vi "RSZVB Set Generator Step Attenuators.vi"(7 "Attenuation Factor (0.0)":dbl format="%^.3e", 8 "error in (no error)":errorcluster {"code" format="%.0x"}, 9 "Port (1)":i32=1, 10 "Channel (1)":i32=1, 11 "VISA session":refnum<visa-resource-name>) -> (0 "error out":errorcluster {"code" format="%.0x"}, 3 "dup VISA session":refnum<visa-resource-name>)   [LabVIEW 2011]
doc: "This VI sets a fixed attenuation factor for the generated wave at test port no. <Pt>. \n\nNote(s):\n\n(1) This VI can be used only with R&S ZVA and ZVB instruments.\n\nRemote-control command(s):\nSOURce<Ch>:POWer<Pt>:ATTenuation <numeric_value>"
uses:
  _utility/RSZVB Global Data.vi
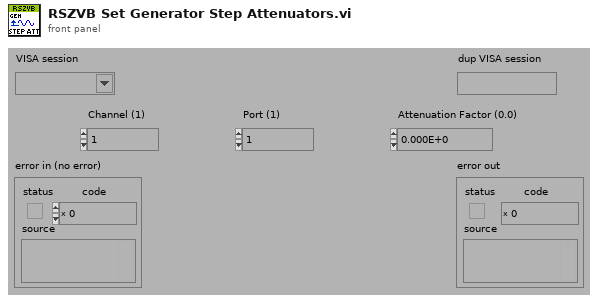
[diagram p1: front panel]
types:
  T1 = cluster{"Error Checking (T: On)":bool, "Installed Options":string[], "Data Valid?":bool, "Ports":i32, "Model":string[], "Option Checking (T: On)":bool}[]
  T2 = cluster{"Error Checking (T: On)":bool, "Installed Options":string[], "Data Valid?":bool, "Ports":i32, "Model":string[], "Option Checking (T: On)":bool}
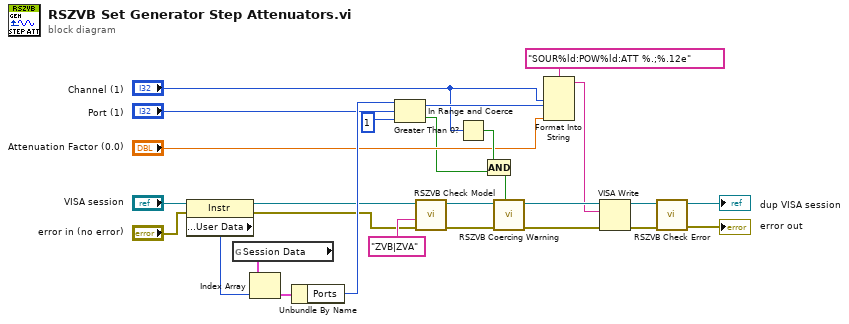
[diagram p0: block diagram]
diagram:
  n1 = property class="Instr"(reference="VISA session", error in="error in (no error)") -> (reference out=w9:refnum<visa-resource-name>, error out=w8:errorcluster, "General Settings:User Data"=w14:u32)
  n2 = global read "RSZVB Global Data.vi" "Session Data"() -> (w15:T1)
  n3 = Index Array(array=w15, index=w14) -> (element=w16:T2)
  n4 = Unbundle By Name(w16) -> ("Ports"=w13:i32)
  n5 = In Range and Coerce(upper limit=w13, x="Port (1)", lower limit=1) -> (coerced(x)=w5:i32, In Range?=w6:bool)
  n6 = call "RSZVB Check Model.vi"("error in (no error)"=w8, "Model"="ZVB|ZVA" ("Options"), "VISA session"=w9) -> ("error out"=w19:errorcluster, "dup VISA session"=w18:refnum<visa-resource-name>)  [unwired: 7 in]
  n7 = Greater Than 0?(x="Channel (1)") -> (x > 0?=w20:bool)
  n8 = Compound Arithmetic op=AND(w20, w6) -> (w22:bool)
  n9 = call "RSZVB Coercing Warning.vi"("In Range?"=w22, "error in (no error)"=w19, "VISA session"=w18) -> ("error out"=w25:errorcluster, "dup VISA session"=w26:refnum<visa-resource-name>)  [unwired: 7 in]
  n10 = Format Into String(format string="SOUR%ld:POW%ld:ATT %.;%.12e", "Channel (1)", w5, "Attenuation Factor (0.0)") -> (resulting string=w21:string)  [unwired: 2 in, 1 out]
  n11 = VISA Write(VISA resource name=w26, write buffer=w21, error in (no error)=w25) -> (VISA resource name out=w23:refnum<visa-resource-name>, error out=w24:errorcluster)  [unwired: 1 out]
  n12 = call "RSZVB Check Error.vi"("error in (no error)"=w24, "VISA session"=w23) -> ("error out"=→"error out":errorcluster, "dup VISA session"=→"dup VISA session":refnum<visa-resource-name>)  [unwired: 8 in]
